vi "Power Off.vi"(8 "error in":errorcluster, 11 "PowerSupply in":refnum<class "PowerSupply.lvclass">) -> (0 "error out":errorcluster, 3 "PowerSupply out":refnum<class "PowerSupply.lvclass">)   [LabVIEW 2019, in "PowerSupply.lvlib" / "PowerSupply.lvclass"]
uses:
  Library/PowerSupply.lvclass
  Library/PowerSupply.lvclass/PowerSupply.ctl
  Accessors/Write Active Channel.vi
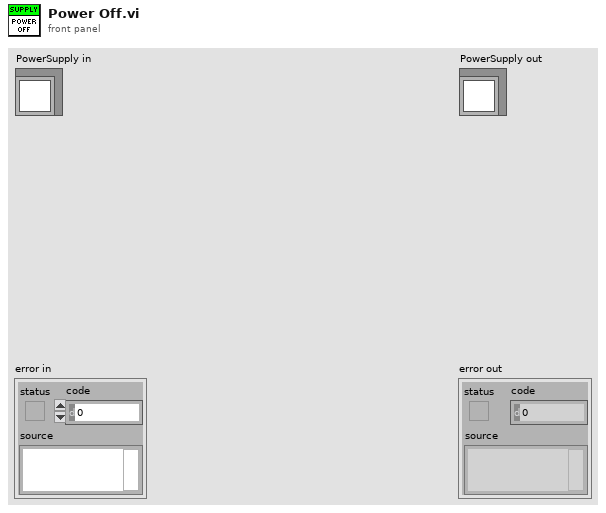
[diagram p1: front panel]
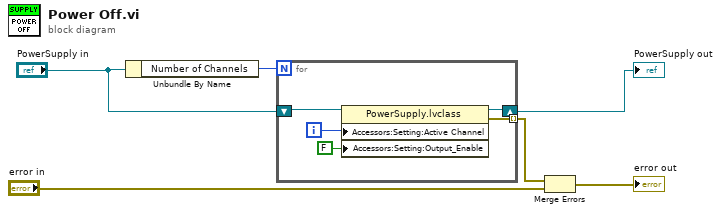
[diagram p0: block diagram]
diagram:
  n1 = Unbundle By Name("PowerSupply in") -> ("Number of Channels"=w6:i32)
  n2 = for {
    N: w6 -> [_]
    shift-right: [w10] -> w4
    shift-left: "PowerSupply in" -> [w11]
    tunnel: [w7] -> w3 mode=indexing
    i -> [w9]
    n3 = property class="PowerSupply.lvclass"(reference=w11, "Accessors:Setting:Active Channel"=w9, "Accessors:Setting:Output_Enable"=FALSE ("Supply:Settings:Output_Enable")) -> (reference out=w10:refnum<class "PowerSupply.lvclass">, error out=w7:errorcluster)  [unwired: 1 in]
  }
  "PowerSupply out" <- w4
  n4 = Merge Errors(w3, "error in") -> (→"error out":errorcluster)
